vi "PH_AxisGUI_NF2.constructor.vi"(0 "name":string, 2 "data in":string, 5 "error in(no error)":errorcluster) -> (14 "i ref out":refnum<vi>, 16 "data out":string, 19 "error out":errorcluster)   [LabVIEW 2014, in "PH_AxisGUI_NF2.lvlib"]
doc: "This class is forseen to control up to three New Focus motors (class: NF87xx).\n\nThis class is part of the PHELIX user layer.\n\nauthor: Stefan Götte, GSI\n\nLicense Agreement for this software:\n\nCopyright (C)\nGesellschaft für Schwerionenforschung, GSI\nPlanckstr. 1\n64291 Darmstadt\nGermany\n\nContact: D.Beck@gsi.de \n\nThis program is free software; you can redistribute it and/or modify it under the terms of the \nGNU General Public License as published by the Free Software Foundation; either version 2 of \nthe license, or (at your option) any later version.\n\nThis program is distributed in the hope that it will be useful, but WITHOUT ANY WARRANTY; \nwithout even the implied warranty of MERCHANTABILITY or FITNESS FOR A PARTICULAR PURPOSE. See the GNU General License for more details (http://www.gnu.org).\n\nGesellschaft für Schwerionenforschung, GSI\nPlanckstr. 1, 64291 Darmstadt, Germany\nFor all questions and ideas contact: M.Richter@gsi.de, H.Brand@gsi.de or D.Beck@gsi.de.\nLast update: 16-JUN-2004"
uses:
  PH_AxisGUI_NF2.lvlib
  CS_Core/CSObj/CSObj.lvlib
  PH_Basics/PH_Class/PH_Class.lvlib
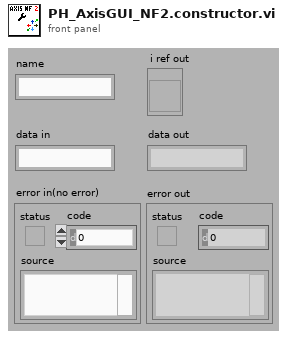
[diagram p1: front panel]
types:
  T1 = enum16{"SetAttribute", "GetAttribute", "CreateAttribute", "DestroyAttribute", "DestroyAllAtributes"}
  T2 = typedef "PH_AxisGUI_NF2.lvlib/PH_AxisGUI_NF2.i attribute.ctl" = cluster{"GUI Refs":cluster{"Delete":refnum<vi>, "Instance Status":refnum<vi>, "Width Axis 1":refnum<vi>, "Width Axis 2":refnum<vi>}, "Instance":string, "System":string, "Width Axis 1":i32, "Width Axis 2":i32, "Sign Change Axis 1":bool, "Sign Change Axis 2":bool, "Motor Axis 1":i32, "Motor Axis 2":i32}
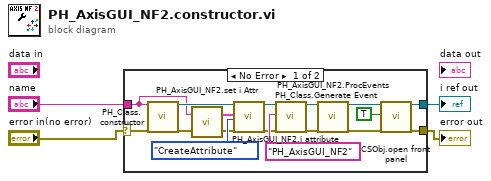
[diagram p0: block diagram]
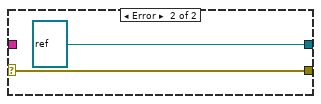
[diagram p2: hidden frame]
diagram:
  n1 = case shown="No Error" "error in(no error)" {
    selector: "error in(no error)" -> [w17 w23]
    tunnel: "name" -> [w5 _]
    tunnel: [w19 refnum<vi> refnum ("i ref out")] -> w3
    tunnel: [w18 w23] -> w2
    frame No Error {
      n2 = call "PH_Class.constructor.vi"("name"=w5, "error in"=w17) -> ("i ref out"=w6:refnum<vi>, "error out"=w11:errorcluster)  [unwired: 15 in, 1 out]
      n3 = call "PH_AxisGUI_NF2.set i Attr.vi"("error in (no error)"=w11, "DB Entry to read"=w5) -> ("error out"=w9:errorcluster, "i Attributes"=w10:T2)
      n4 = call "PH_AxisGUI_NF2.i attribute.vi"("VI Refnum"=w6, "CLASS.i attribute"=w10, "Action"=T1."CreateAttribute", "error in (no error)"=w9) -> ("VI Refnum out"=w8:refnum<vi>, "error out"=w7:errorcluster)  [unwired: 13 in, 1 out]
      n5 = call "PH_Class.Generate Event.vi"("i ref in"=w8, "Class"="PH_AxisGUI_NF2", "error in (no error)"=w7) -> ("i ref out"=w16:refnum<vi>, "error out"=w15:errorcluster)  [unwired: 15 in]
      n6 = call "PH_AxisGUI_NF2.ProcEvents.vi"("i ref in"=w16, "error in"=w15) -> ("i ref out"=w14:refnum<vi>, "error out"=w13:errorcluster)  [unwired: 16 in]
      n7 = call "CSObj.open front panel.vi"("i ref in"=w14, "frontPanelOpen"=TRUE ("front panel open"), "error in (no error)"=w13) -> ("i ref out"=w19:refnum<vi>, "error out"=w18:errorcluster)  [unwired: 15 in]
    }
    frame Error {
    }
  }
  "i ref out" <- w3
  "error out" <- w2
